vi "Read Control Metadata.vi"(8 "error in":errorcluster, 11 "Value in":refnum<class "Value.lvclass">) -> (0 "error out":errorcluster, 1 "has control metadata?":bool, 2 "control metadata":T1, 3 "Value out":refnum<class "Value.lvclass">)   [LabVIEW 2020, in "Value.lvlib" / "Value.lvclass"]
uses:
  Value.lvclass
  Control Metadata.ctl
  Value.lvlib
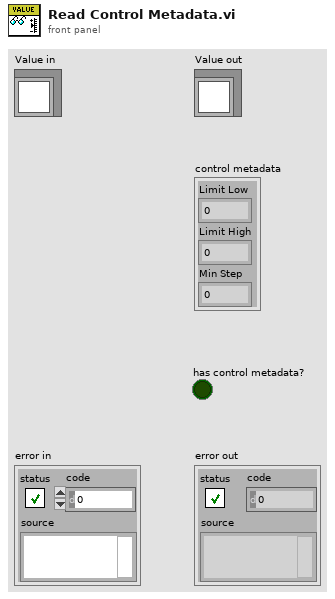
[diagram p1: front panel]
types:
  T1 = typedef "Value.lvlib/Control Metadata.ctl" = cluster{"Limit Low":dbl, "Limit High":dbl, "Min Step":dbl}
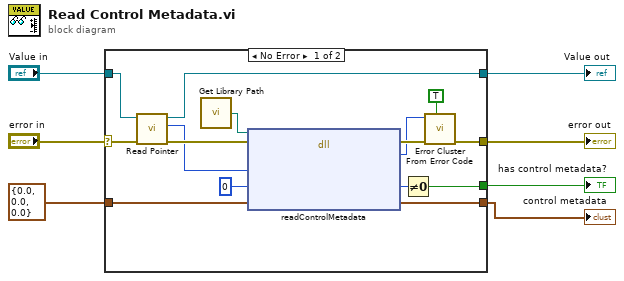
[diagram p0: block diagram]
diagram:
  n1 = case shown="No Error" "error in" {
    selector: "error in" -> [w17 w24]
    tunnel: [w18 w24] -> w7
    tunnel: "Value in" -> [w15 w23]
    tunnel: [w13 w23] -> w4
    tunnel: T1 {"Limit Low"=0.0, "Limit High"=0.0, "Min Step"=0.0} ("Control Metadata") -> [w12 _]
    tunnel: [w9 _] -> w3
    tunnel: [w8 _] -> w2
    frame No Error {
      n2 = call-dynamic "Read Pointer.vi"("error in (no error)"=w17, "Value in"=w15) -> ("error out"=w16:errorcluster, "pointer"=w14:i64, "Value out"=w13:refnum<class "Value.lvclass">)  [unwired: 7 in]
      n3 = call "Get Library Path.vi"() -> ("Path"=w22:path)  [unwired: 1 in]
      n4 = dll-call lib="?" fn="readControlMetadata"(path in=w22, error in=w16, "value"=w14, "has control metadata?"=i16 0 ("has display metadata?"), "control metadata"=w12) -> (error out=w20:errorcluster, "err_code"=w19:i32, "has control metadata?"=w11:i16, "control metadata"=w8:T1)  [unwired: 2 in, 1 out]
      n5 = Not Equal To 0?(x=w11) -> (x != 0?=w9:bool)
      n6 = call <vilib>:"Error Cluster From Error Code.vi"("show call chain? (False)"=TRUE, "error in (no error)"=w20, "error code (0)"=w19) -> ("error out"=w18:errorcluster)  [unwired: 6 in]
    }
    frame Error {
    }
  }
  "error out" <- w7
  "Value out" <- w4
  "has control metadata?" <- w3
  "control metadata" <- w2
